vi "st_Geometric PDF (kx).vi"(10 "p":dbl=0.5, 11 "x":dbl=1.0) -> (0 "error":i32, 3 "pdf(x)":dbl=0.25)   [LabVIEW 2010, in "NI_Gmath.lvlib"]
uses:
  NI_Gmath.lvlib
  st_error_code.ctl
panel:
  # "Geometric PDF"
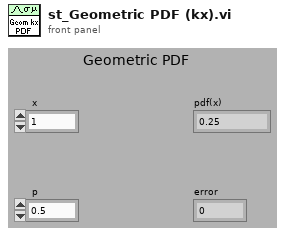
[diagram p1: front panel]
types:
  T1 = typedef "NI_Gmath.lvlib/st_error_code.ctl" = i32
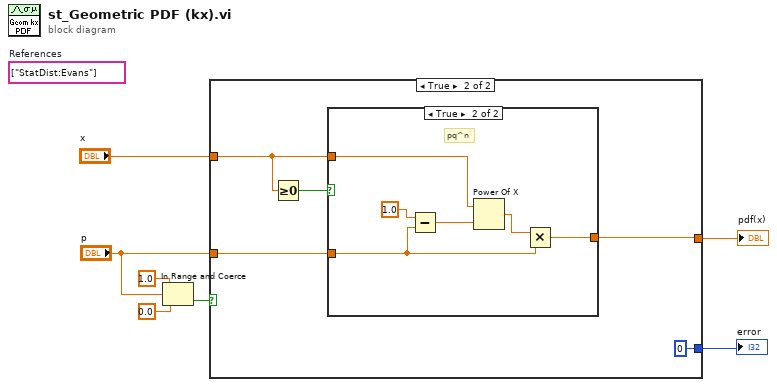
[diagram p0: block diagram]
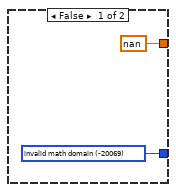
[diagram p2: hidden frame]
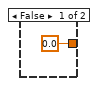
[diagram p3: hidden frame]
diagram:
  (unwired) string[] ["StatDist:Evans"]  # References
  n1 = In Range and Coerce(upper limit=1.0, x="p", lower limit=0.0) -> (In Range?=w4:bool)  [unwired: 1 out]
  n2 = case shown="True" w4 {
    tunnel: [w8 0 ("invalid math domain")] -> w7
    tunnel: [nan w12] -> w6
    tunnel: "x" -> [_ w10]
    tunnel: "p" -> [_ w11]
    frame False {
      w8 = T1 -20069 items=["invalid math domain"=-20069, "Fourier interpolation size m >= n"=-20070, "empty array"=-20003] ("stat interp error code")
    }
    frame True {
      n3 = Greater Or Equal To 0?(x=w10) -> (x >= 0?=w13:bool)
      n4 = case shown="True" w13 {
        tunnel: [0.0 w17] -> w12
        tunnel: w11 -> [_ w16]
        tunnel: w10 -> [_ w19]
        frame False {
        }
        frame True {
          # "pq^n"
          n5 = Subtract(x=1.0, y=w16) -> (x-y=w20:dbl)
          n6 = Power Of X(1:w20, 2:w19) -> (0:w18:dbl)
          n7 = Multiply(x=w18, y=w16) -> (x*y=w17:dbl)
        }
      }
    }
  }
  "pdf(x)" <- w6
  "error" <- w7
